vi "Test01_Utilities.vi"() -> ()   [LabVIEW 2018]
panel:
  out "Error Out":errorcluster
  in  "Error In":errorcluster
  out "error_code":i32
  in  "device_id":i32
  out "error_code":i32
  out "error_code":i32
  in  "device_id":i32
  out "error_code":i32
  out "Num CUDA Devices":i32
  out "Error Codes":string
  out "GPU Info":string
  # "GPU CUDA -"
  # "UTILITIES"
  # "Get CUDA Devices"
  # "Reset Device"
  # "Reset All Devices"
  # "Set Device"
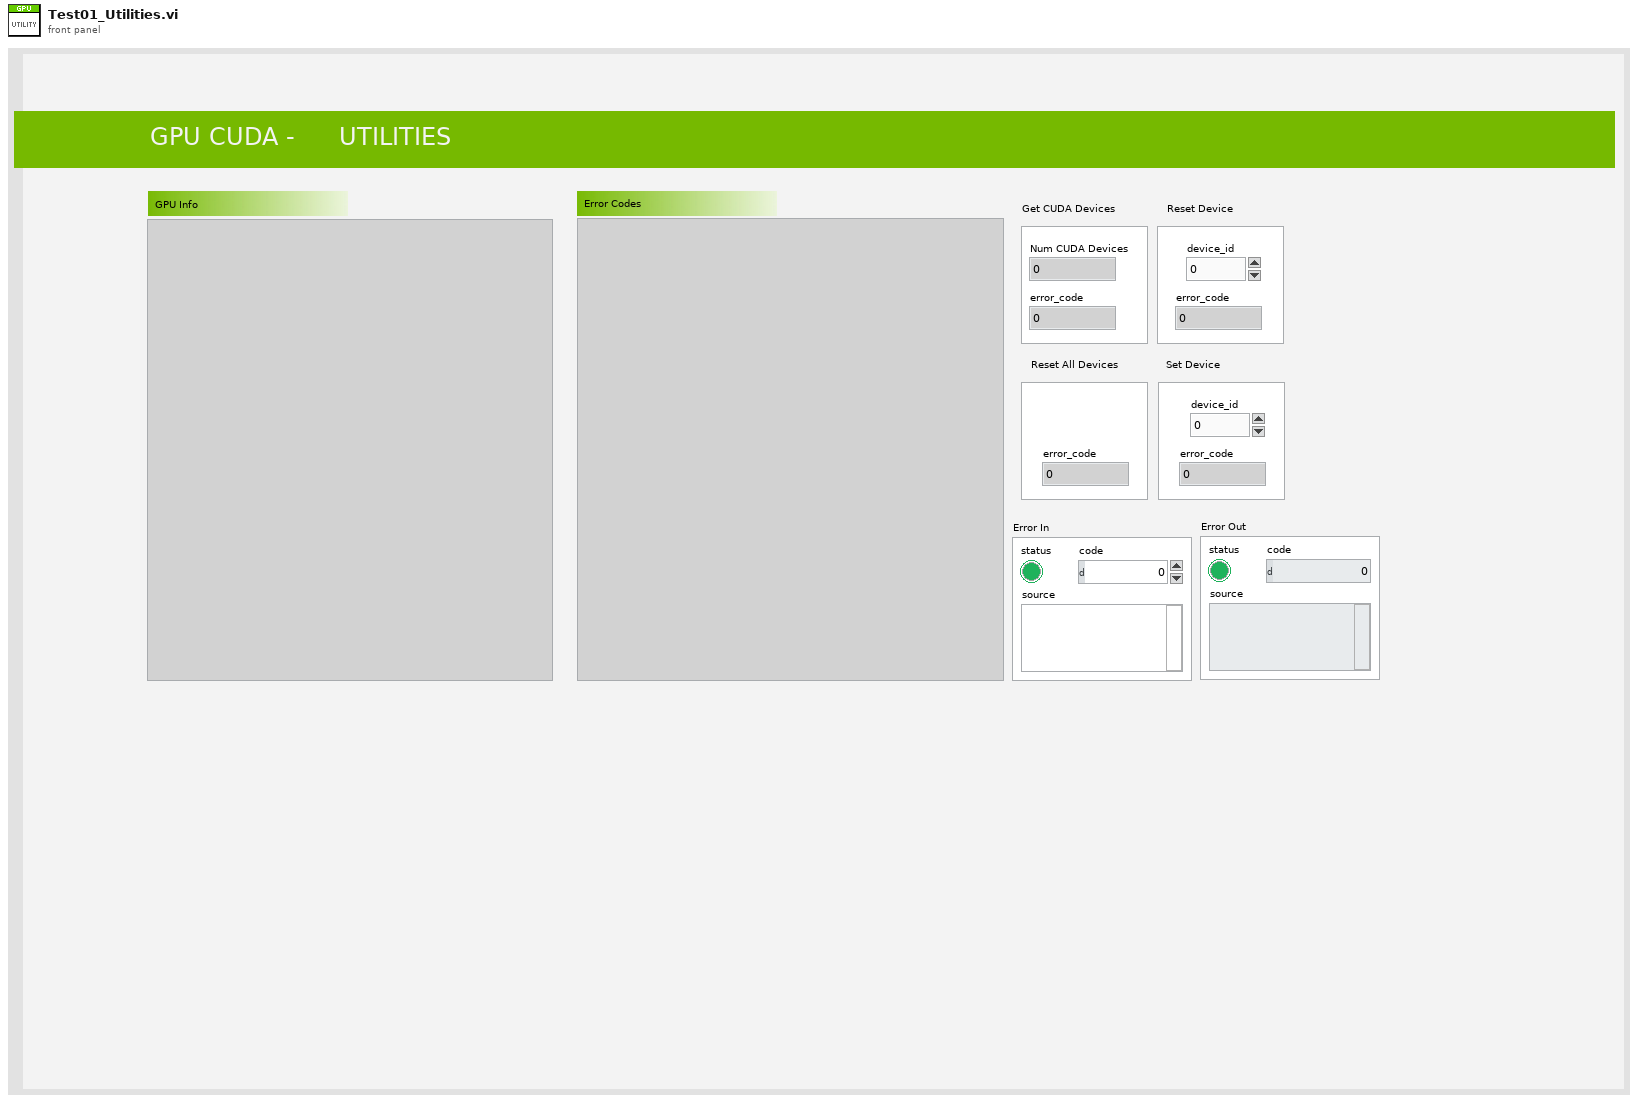
[diagram p1: front panel]
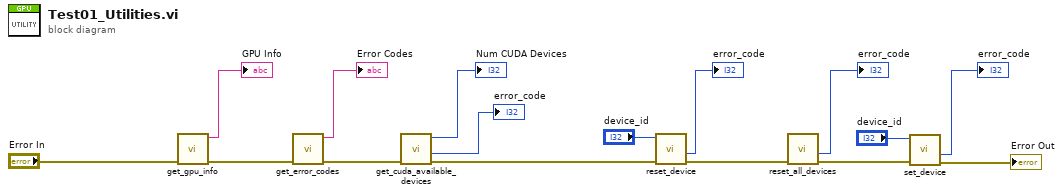
[diagram p0: block diagram]
diagram:
  n1 = call "get_gpu_info.vi"("Error in"="Error In") -> ("Error out"=w15:errorcluster, "GPU Info"=→"GPU Info":string)  [unwired: 9 in]
  n2 = call "get_error_codes.vi"("Error in 2"=w15) -> ("Error out 2"=w13:errorcluster, "Error Codes"=→"Error Codes":string)  [unwired: 9 in]
  n3 = call "get_cuda_available_devices.vi"("Error in"=w13) -> ("Error out"=w10:errorcluster, "error_code"=→"error_code":i32, "num_cuda_devices"=→"Num CUDA Devices":i32)  [unwired: 8 in]
  n4 = call "reset_device.vi"("Error in"=w10, "device_id"="device_id") -> ("Error out"=w9:errorcluster, "error_code"=→"error_code":i32)  [unwired: 8 in]
  n5 = call "reset_all_devices.vi"("Error in"=w9) -> ("Error out"=w8:errorcluster, "error_code"=→"error_code":i32)  [unwired: 9 in]
  n6 = call "set_device.vi"("Error in"=w8, "device_id 2"="device_id") -> ("Error out"=→"Error Out":errorcluster, "error_code"=→"error_code":i32)  [unwired: 8 in]
